vi "sendOnQueue.vi"(8 "error in (no error)":errorcluster, 9 "Message In":string, 10 "Queue Name in":string, 11 "RabbitMQ Session In":T1) -> (0 "error out":errorcluster, 1 "Message out":string, 2 "Queue Name out":string, 3 "RabbitMQ Session Out":T1)   [LabVIEW 2019, in "rabbitmq.lvlib"]
uses:
  session.ctl
  rabbitmq.lvlib
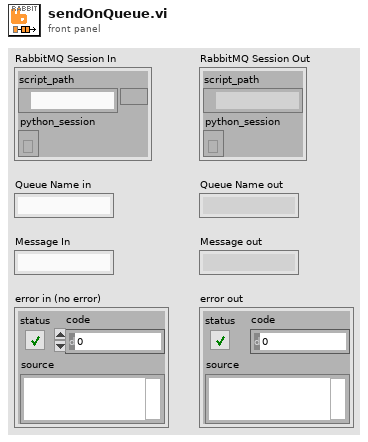
[diagram p1: front panel]
types:
  T1 = typedef "rabbitmq.lvlib/session.ctl" = cluster{"script_path":path, "python_session":refnum<k35>}
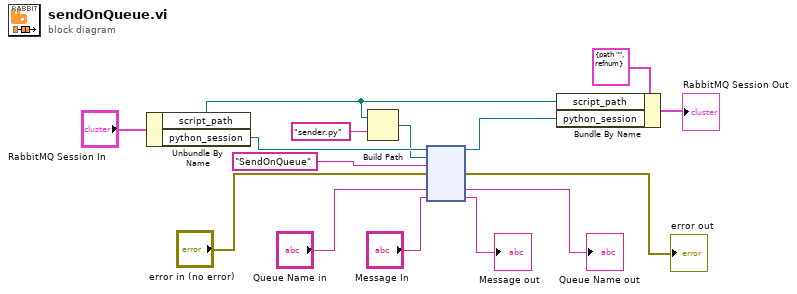
[diagram p0: block diagram]
diagram:
  n1 = Unbundle By Name("RabbitMQ Session In") -> ("script_path"=w2:path, "python_session"=w8:refnum<k35>)
  n2 = Build Path(base path=w2, name or relative path="sender.py") -> (appended path=w1:path)
  n3 = node(w8, w1, "SendOnQueue" ("function name"), "error in (no error)", "Queue Name in", "Message In") -> (w15:refnum<k35>, →"error out":errorcluster, →"Queue Name out":string, →"Message out":string)  [unwired: 2 in, 2 out]
  n4 = Bundle By Name(cluster=T1 {"script_path"=path "", "python_session"=refnum}, "script_path"=w2, "python_session"=w15) -> (→"RabbitMQ Session Out":T1)
